vi "Get Python Version.vi"() -> (2 "Python String":string)   [LabVIEW 2021, in "Fixture.lvclass"]
uses:
  Fixture.lvclass
  <vilib>/JDP Science/JDP Science Common Utilities/JDP Utility.lvlib
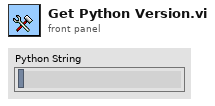
[diagram p1: front panel]
types:
  T1 = typedef "File Paths.ctl" = cluster{"Glue Pattern Folder":path, "Carrier Tray Folder":path, "Pick Up Tool Fixture Folder":path, "Components Folder":path, "Bellows Tool Offset.txt":path, "Pick Up Tool Offset.txt":path, "Dispense Tip Offset.txt":path, "Log Files":path, "Gantry Assembly Map.txt":path, "Syringe and offset map.txt":path, "I_O Pin Map":path, "Controllers":path, "Python DB Conn":path}
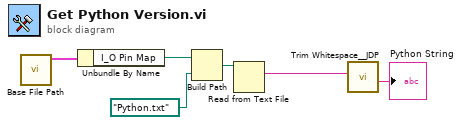
[diagram p0: block diagram]
diagram:
  n1 = call "Base File Path.vi"() -> ("Paths Out"=w6:T1)  [unwired: 11 in]
  n2 = Unbundle By Name(w6) -> ("I_O Pin Map"=w5:path)
  n3 = Build Path(base path=w5, name or relative path=path "Python.txt") -> (appended path=w3:path)
  n4 = Read from Text File(file (use dialog)=w3) -> (text=w2:string)  [unwired: 3 in, 3 out]
  n5 = call <vilib>:"Trim Whitespace__JDP.vi"("String in"=w2) -> ("String out"=→"Python String":string)  [unwired: 6 in]
